vi "set_pixel_frequency.vi"(8 "error in (no error)":errorcluster, 10 "pixel frequency":dbl[unit], 11 "FPGAWrapperAN110607Galvo in":refnum<class "FPGAWrapperAN110607Galvo.lvclass">) -> (0 "error out":errorcluster, 3 "FPGAWrapperAN110607Galvo out":refnum<class "FPGAWrapperAN110607Galvo.lvclass">)   [LabVIEW 2010, in "FPGAWrapperAN110607Galvo.lvclass"]
uses:
  FPGAWrapperAN110607Galvo.lvclass
  <vilib>/rvi/interface/nirviReadWriteControl/nirviReadWriteControl.xnode
  FPGA_VI_ref.ctl
  <vilib>/rvi/interface/common/niFpgaNodeNameForErrorReporting.ctl
  <vilib>/rvi/errors/niLvFpgaWhatHappensToTopLevelVI.ctl
  <vilib>/Utility/error.llb/Error Cluster From Error Code.vi
  <vilib>/rvi/errors/niLvFpgaAdjustHostInterfaceError.vi
  NiFpgaLv.dll
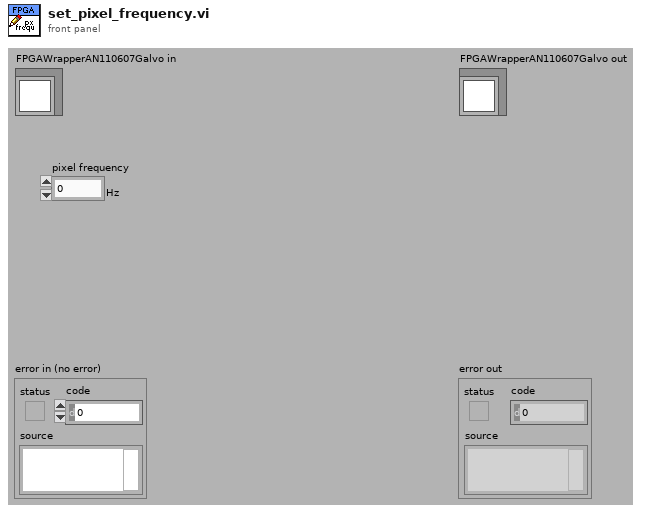
[diagram p1: front panel]
types:
  T1 = typedef "niFpgaNodeNameForErrorReporting.ctl" = enum16{"Open FPGA VI Reference", "Read/Write Control", "Invoke Method: Abort", "Invoke Method: Acknowledge IRQ", "Invoke Method: Download", "Invoke Method: FIFO.Configure", "Invoke Method: FIFO.Read", "Invoke Method: FIFO.Start", "Invoke Method: FIFO.Stop", "Invoke Method: FIFO.Write", "Invoke Method: Reset", "Invoke Method: Run", "Invoke Method: Wait on IRQ", "Close FPGA VI Reference"}
  T2 = typedef "niLvFpgaWhatHappensToTopLevelVI.ctl" = enum16{"top level VI scripted behind XNode", "top level VI inlined behind XNode"}
  T3 = typedef "FPGAWrapperAN110607Galvo.lvclass/FPGA_VI_ref.ctl" = refnum<k20>
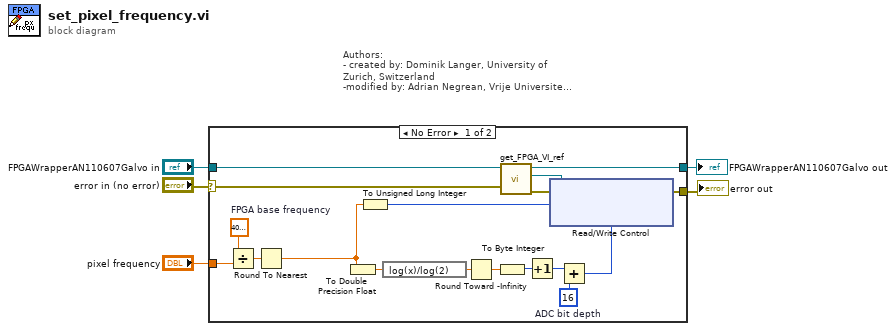
[diagram p0: block diagram]
diagram:
  n1 = case "Authors: \n- created by: Dominik Langer, University of Zurich, Switzerland\n-modified by: Adrian Negrean, Vrije Universiteit Amsterdam" shown="No Error" "error in (no error)" {
    selector: "error in (no error)" -> [w14 w83]
    tunnel: "FPGAWrapperAN110607Galvo in" -> [w15 w84]
    tunnel: [w12 w84] -> w3
    tunnel: [w23 w83] -> w4
    tunnel: "pixel frequency" -> [w9 _]
    frame No Error {
      w8 = dbl[unit] 40000000.0  # FPGA base frequency
      w20 = i8 16  # ADC bit depth
      n2 = Divide(x=w8, y=w9) -> (x/y=w7:dbl)
      n3 = Round To Nearest(number=w7) -> (nearest integer value=w6:dbl)
      n4 = To Double Precision Float(number=w6) -> (double precision float=w18:dbl)
      n5 = To Unsigned Long Integer(number=w6) -> (unsigned 32bit integer=w22:u32)
      n6 = expression code="log(x)/log(2)"(w18) -> (w17:dbl)
      n7 = Round Toward -Infinity(1:w17) -> (0:w21:dbl)
      n8 = To Byte Integer(number=w21) -> (8bit integer=w19:i8)
      n9 = call-dynamic "get_FPGA_VI_ref.vi"("error in (no error)"=w14, "FPGAWrapperAN110607Galvo in"=w15) -> ("error out"=w13:errorcluster, "FPGA VI reference"=w16:T3, "FPGAWrapperAN110607Galvo out"=w12:refnum<class "FPGAWrapperAN110607Galvo.lvclass">)  [unwired: 7 in]
      n10 = Increment(x=w19) -> (x+1=w10:i8)
      n11 = Add(x=w10, y=w20) -> (x+y=w11:i8)
      n12 = xnode "Read/Write Control"("FPGA VI Reference In"=w16, "error in"=w13, "iterations per pixel"=w22, "maximum bit depth"=w11) -> ("error out"=w23:errorcluster)  [unwired: 1 out]
    }
    frame Error {
    }
  }
  "error out" <- w4
  "FPGAWrapperAN110607Galvo out" <- w3
